vi "Vocht To HTML Improovd.vi"(0 "vochtigheid 4":refnum<vi>, 1 "path to JPEG file":path) -> ()   [LabVIEW 2013]
panel:
  out "vochtigheid 3":i32[](graph)
  out "vochtigheid 2":i32[](graph)
  in  "vochtigheid":i32[](graph)
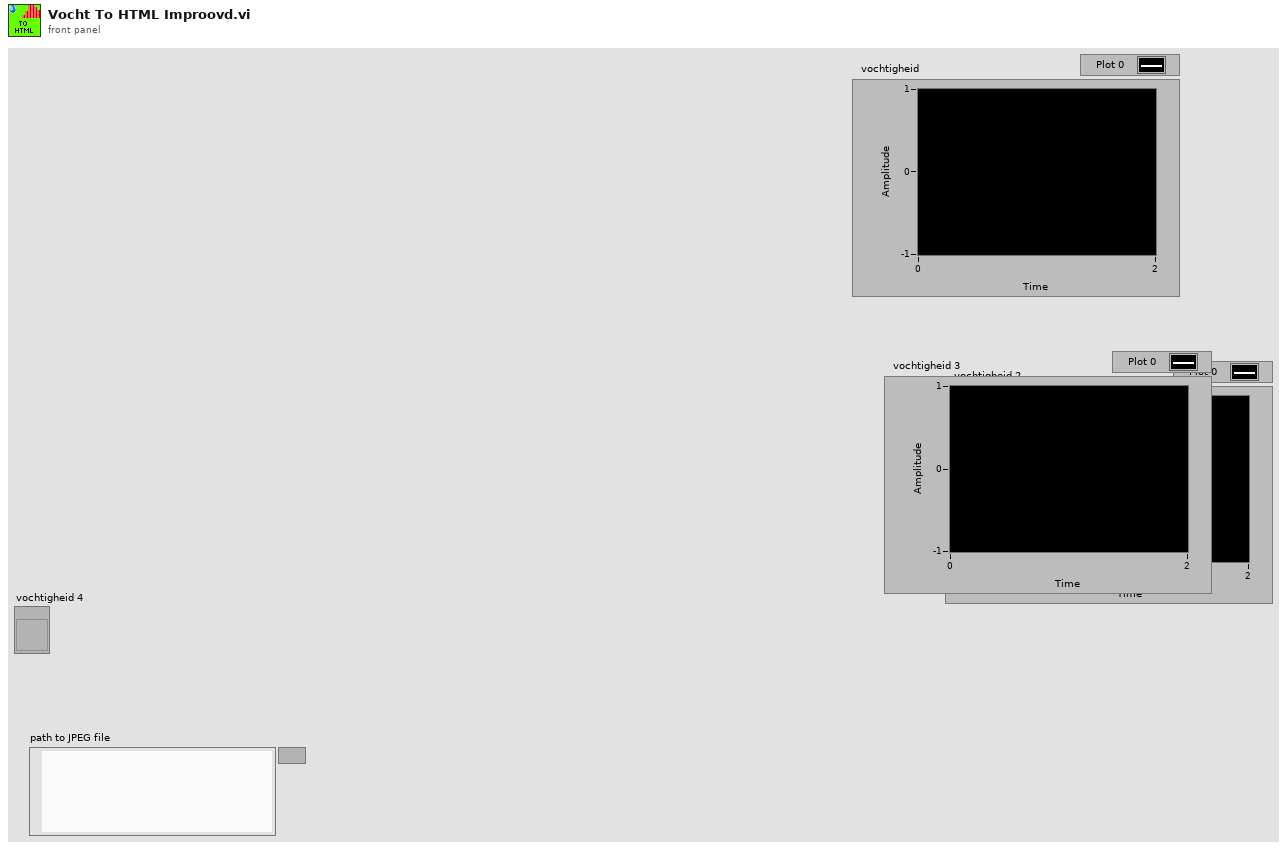
[diagram p1: front panel]
types:
  T1 = typedef "imagedata.ctl" = cluster{"image type":i32, "image depth":i32, "image":u8[], "mask":u8[], "colors":u32[], "Rectangle":cluster{"left":i16, "top":i16, "right":i16, "bottom":i16}}
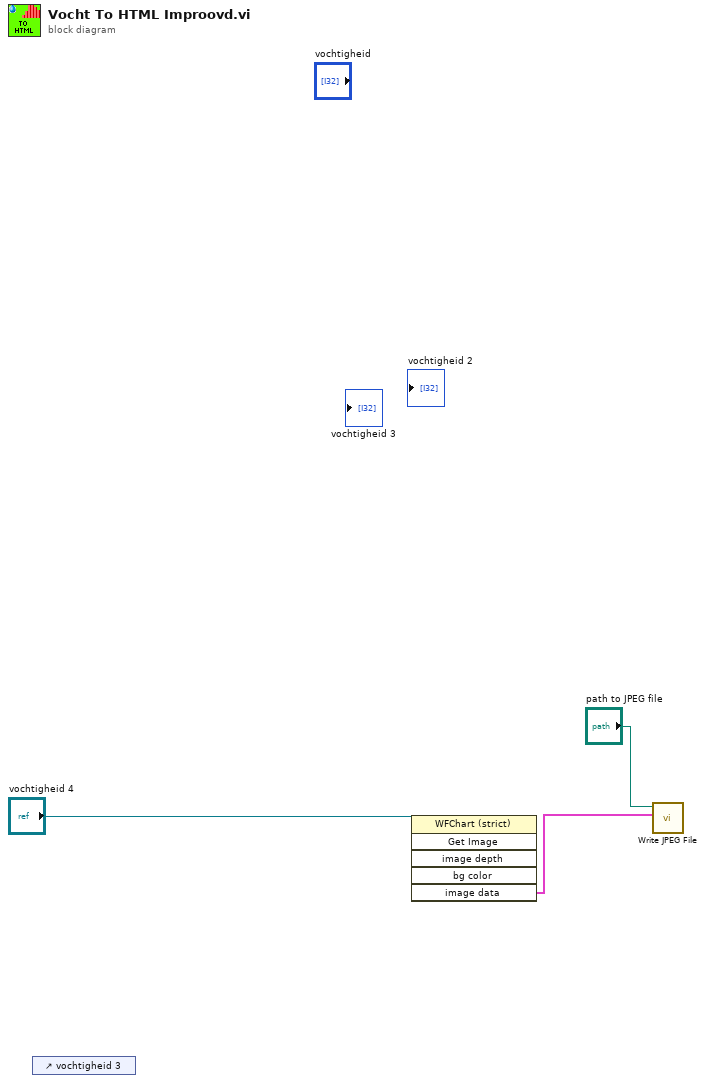
[diagram p0: block diagram]
diagram:
  n1 = control-ref of="vochtigheid 3"() -> ()  [unwired: 1 out]
  n2 = invoke on="Invoke Node" class="WFChart (strict)" method="Get Image"(reference="vochtigheid 4") -> ("image data"=w2:T1)  [unwired: 5 in, 5 out]
  n3 = call <vilib>:"Write JPEG File.vi"("image data"=w2, "path to JPEG file"="path to JPEG file") -> ()  [unwired: 8 in, 2 out]
